vi "Proj3_Wireless_DTMF_Receiver.vi"(0 "Ringtone Path":path=path "C:/Users/Sungeun/Dropbox/Lab/DTMF/VI Source/Project 3/ringtone/Nokia_Original.wav", 4 "Gray Bit Encoding":bool, 6 "Quantization Level":u16(ring)=4 items=["2"=2, "4"=4, "8"=8, "16"=16], 8 "Ringtone":bool, 9 "My Phone Number":string, 11 "RXbitStream":i8[](array[numeric]) min=0 max=1) -> (1 "Received Digits":string, 3 "dequants":dbl[](array[numeric]))   [LabVIEW 2011]
panel:
  in  "stop? (T)":bool
  out "Received Quantized DTMF Signal":dbl[](graph)
  in  "bitLength":i32
  in  "Tab Control":enum32{"DTMF", "Quantization"}(tab)
  # "Project 3: Wireless DTMF Receiver"
  # "Receiver"
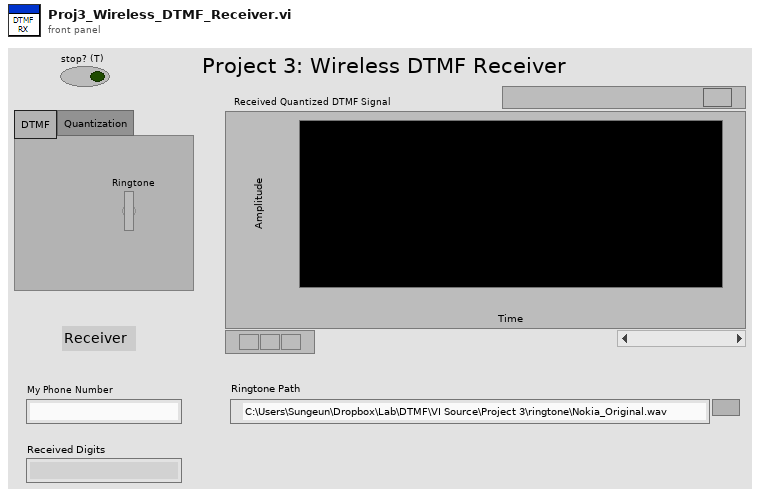
[diagram p1: front panel]
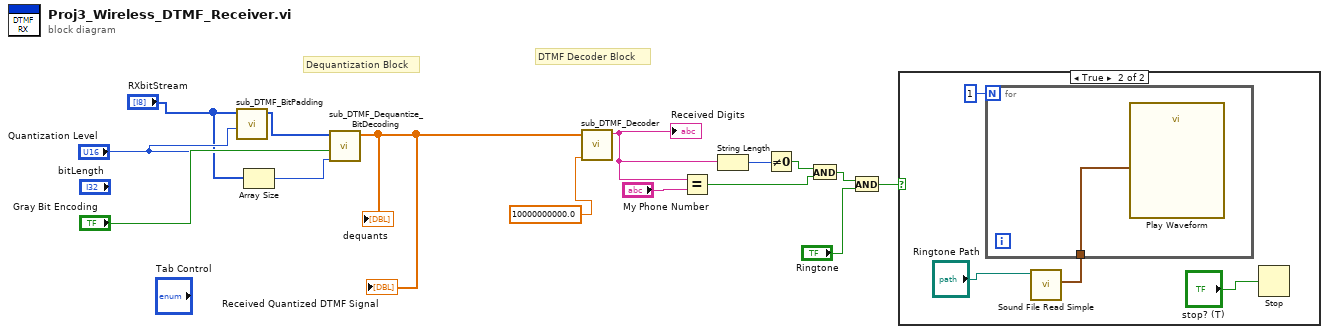
[diagram p0: block diagram]
diagram:
  # "DTMF Decoder Block"
  # "Dequantization Block"
  n1 = call "sub_DTMF_BitPadding.vi"("Modulation Order"="Quantization Level", "TXbitStream"="RXbitStream") -> ("TXbitStream Output"=w3:i8[])  [unwired: 8 in, 1 out]
  n2 = Array Size(array="RXbitStream") -> (size(s)=w2:i32)
  n3 = call "sub_DTMF_Dequantize_BitDecoding.vi"("bitLength"=w2, "GrayCode"="Gray Bit Encoding", "L"="Quantization Level", "RXbitStream"=w3) -> ("dequants"=w13:dbl[])  [unwired: 7 in]
  "Received Quantized DTMF Signal" <- w13
  "dequants" <- w13
  n4 = call "sub_DTMF_Decoder.vi"("SNRdB"=10000000000.0, "signal"=w13) -> ("digits"=w11:string)  [unwired: 9 in]
  "Received Digits" <- w11
  n5 = Equal?(x=w11, y="My Phone Number") -> (x = y?=w8:bool)
  n6 = String Length(string=w11) -> (length=w10:i32)
  n7 = Not Equal To 0?(x=w10) -> (x != 0?=w9:bool)
  n8 = And(x=w9, y=w8) -> (x .and. y?=w7:bool)
  n9 = And(x=w7, y="Ringtone") -> (x .and. y?=w6:bool)
  n10 = case shown="True" w6 {
    frame False {
    }
    frame True {
      n11 = call <vilib>:"Sound File Read Simple.vi"("path"="Ringtone Path") -> ("data"=w18:waveform(dbl)[])  [unwired: 7 in, 3 out]
      n12 = for {
        N: 1 -> [_]
        tunnel: w18 -> [w20]
        n13 = call "Play Waveform"("Data"=w20) -> ()  [unwired: 18 in, 1 out]
      }
      n14 = Stop(stop? (T)="stop? (T)") -> ()
    }
  }
